vi "Lockin.Low Pass Filter Bank.vi"(6 "Butterworth? [T]":bool=TRUE, 8 "error in (no error)":errorcluster, 10 "WFms in":waveform(dbl)[](array[waveform]), 11 "DSP in":refnum<class "DSP.lvclass">) -> (0 "error out":errorcluster, 2 "Wfms out":waveform(dbl)[](array[waveform]))   [LabVIEW 2019, in "DSP.lvclass"]
uses:
  DSP.lvclass
  Waveform.Attributes/Waveform.Attributes.lvlib
panel:
  out "appended array":errorcluster[](array[cluster])
  out "DSP out":refnum<class "DSP.lvclass">
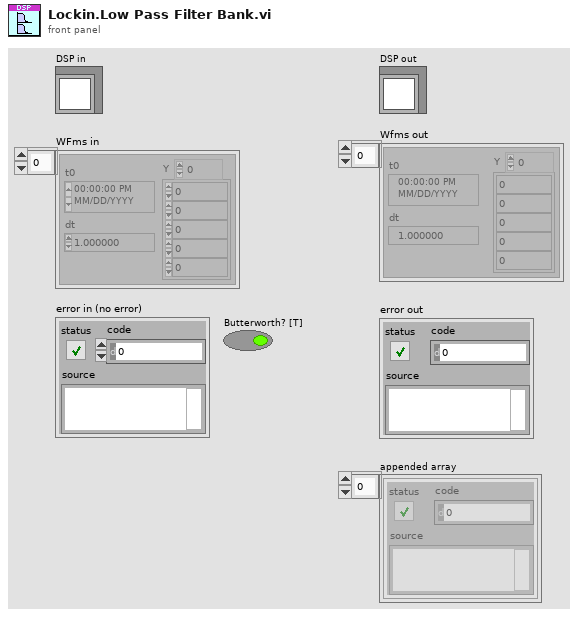
[diagram p1: front panel]
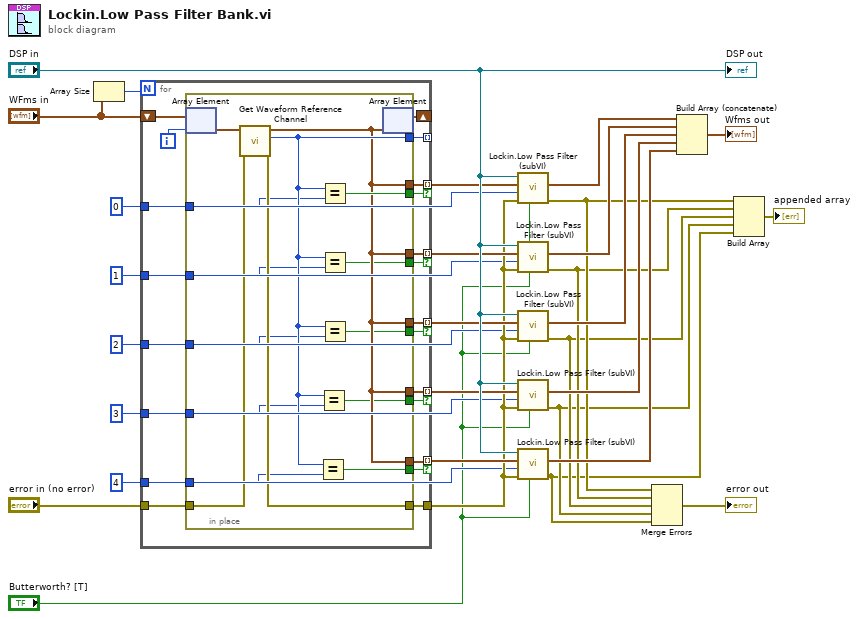
[diagram p0: block diagram]
diagram:
  w12 = 4 ("y")
  w11 = 3 ("y")
  w10 = 2 ("y")
  w9 = 1 ("y")
  w8 = 0 ("y")
  n1 = Array Size(array="WFms in") -> (size(s)=w27:i32)
  n2 = for {
    N: w27 -> [_]
    shift-right: [w45] -> _
    shift-left: "WFms in" -> [w49]
    tunnel: [w46] -> _ mode=indexing
    tunnel: "error in (no error)" -> [w48]
    tunnel: [w47] -> w13
    tunnel: [w44] -> w18 mode=indexing if=w43
    tunnel: [w42] -> w17 mode=indexing if=w35
    tunnel: [w41] -> w16 mode=indexing if=w36
    tunnel: [w40] -> w15 mode=indexing if=w37
    tunnel: [w39] -> w14 mode=indexing if=w38
    tunnel: w12 -> [w34]
    tunnel: w11 -> [w33]
    tunnel: w10 -> [w32]
    tunnel: w9 -> [w31]
    tunnel: w8 -> [w30]
    i -> [w50]
    n3 = in-place {
      in-place-border: w48 -> [w64]
      in-place-border: [w63] -> w47
      in-place-border: [w62] -> w46
      in-place-border: [w60] -> w44
      in-place-border: [w61] -> w43
      in-place-border: [w60] -> w42
      in-place-border: [w60] -> w41
      in-place-border: [w60] -> w40
      in-place-border: [w60] -> w39
      in-place-border: [w59] -> w38
      in-place-border: [w58] -> w37
      in-place-border: [w57] -> w36
      in-place-border: [w56] -> w35
      in-place-border: w34 -> [w55]
      in-place-border: w33 -> [w54]
      in-place-border: w32 -> [w53]
      in-place-border: w31 -> [w52]
      in-place-border: w30 -> [w51]
      n4 = in-place-array #1(w49, w50) -> (w65:waveform(dbl))
      n5 = call "Get Waveform Reference Channel.vi"("error in (no error)"=w64, "Reference in"=w65) -> ("error out"=w63:errorcluster, "Reference Channel"=w62:i32, "Reference out"=w60:waveform(dbl))  [unwired: 7 in]
      n6 = Equal?(x=w62, y=w55) -> (x = y?=w59:bool)
      n7 = Equal?(x=w62, y=w54) -> (x = y?=w58:bool)
      n8 = Equal?(x=w62, y=w51) -> (x = y?=w61:bool)
      n9 = Equal?(x=w62, y=w52) -> (x = y?=w56:bool)
      n10 = Equal?(x=w62, y=w53) -> (x = y?=w57:bool)
      n11 = in-place-array #1(w60) -> (w45:waveform(dbl)[])  [unwired: 1 out]
    }
  }
  n12 = call "Lockin.Low Pass Filter (subVI).vi"("Butterworth? [T]"="Butterworth? [T]", "error in (no error)"=w13, "Element Data"=w8, "signal in"=w18, "DSP in"="DSP in") -> ("error out"=w6:errorcluster, "signal out"=w19:waveform(dbl)[])  [unwired: 3 in, 2 out]
  n13 = call "Lockin.Low Pass Filter (subVI).vi"("Butterworth? [T]"="Butterworth? [T]", "error in (no error)"=w13, "Element Data"=w9, "signal in"=w17, "DSP in"="DSP in") -> ("error out"=w5:errorcluster, "signal out"=w20:waveform(dbl)[])  [unwired: 3 in, 2 out]
  n14 = call "Lockin.Low Pass Filter (subVI).vi"("Butterworth? [T]"="Butterworth? [T]", "error in (no error)"=w13, "Element Data"=w10, "signal in"=w16, "DSP in"="DSP in") -> ("error out"=w4:errorcluster, "signal out"=w21:waveform(dbl)[])  [unwired: 3 in, 2 out]
  n15 = call "Lockin.Low Pass Filter (subVI).vi"("Butterworth? [T]"="Butterworth? [T]", "error in (no error)"=w13, "Element Data"=w11, "signal in"=w15, "DSP in"="DSP in") -> ("error out"=w3:errorcluster, "signal out"=w22:waveform(dbl)[])  [unwired: 3 in, 2 out]
  n16 = call "Lockin.Low Pass Filter (subVI).vi"("Butterworth? [T]"="Butterworth? [T]", "error in (no error)"=w13, "Element Data"=w12, "signal in"=w14, "DSP in"="DSP in") -> ("error out"=w2:errorcluster, "signal out"=w23:waveform(dbl)[])  [unwired: 3 in, 2 out]
  n17 = Merge Errors(w6, w5, w4, w3, w2) -> (→"error out":errorcluster)
  n18 = Build Array (concatenate)(w19, w20, w21, w22, w23) -> (→"Wfms out":waveform(dbl)[])
  n19 = Build Array(w6, w5, w4, w3, w2) -> (→"appended array":errorcluster[])
  "DSP out" <- "DSP in"
